vi "ep_Flicker Aggregation PLT (1ch).vi"(0 "flicker Pst":dbl, 1 "restart (F)":bool, 5 "Pst flicker time":timestamp) -> (4 "flicker Plt":dbl, 6 "Plt flicker time":timestamp, 15 "data valid?":bool)   [LabVIEW 2011, in "NI_EP_Power Quality.lvlib"]
uses:
  <vilib>/addons/Electrical Power/PQ/NI_EP_Power Quality.lvlib
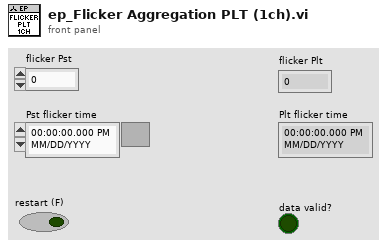
[diagram p1: front panel]
types:
  T1 = typedef "LVDateTimeRec.ctl" = cluster{"fractional second":dbl, "second":i32, "minute":i32, "hour":i32, "day of month":i32, "month":i32, "year":i32, "day of week":i32, "day of year":i32, "DST":i32}
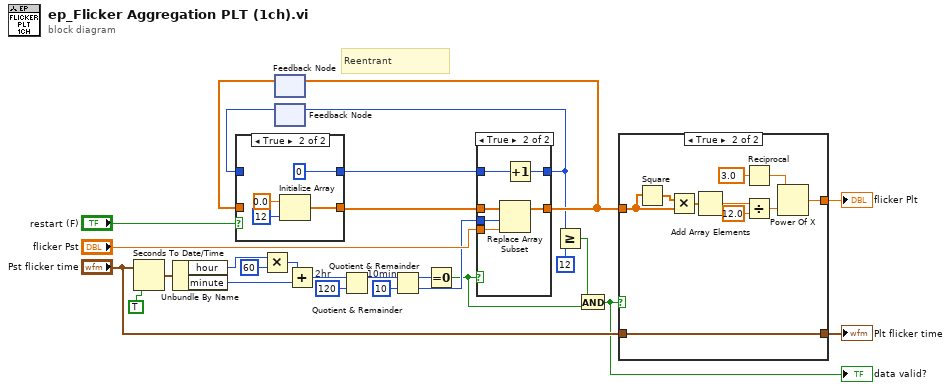
[diagram p0: block diagram]
diagram:
  w15 = 10  # 10min
  w17 = 120  # 2hr
  # "Reentrant"
  n1 = Seconds To Date/Time(time stamp (now)="Pst flicker time", to UTC (F)=TRUE) -> (date time rec=w23:T1)
  n2 = Unbundle By Name(w23) -> ("hour"=w22:i32, "minute"=w19:i32)
  n3 = Multiply(x=w22, y=60) -> (x*y=w20:i32)
  n4 = feedback #1() -> (w26:dbl[])  [unwired: 1 in]
  n5 = feedback #2() -> (w25:i32)  [unwired: 1 in]
  n6 = case shown="True" "restart (F)" {
    tunnel: [w29 w31] -> w12
    tunnel: w26 -> [w29 _]
    tunnel: [w28 0] -> w11
    tunnel: w25 -> [w28 _]
    frame False {
    }
    frame True {
      n7 = Initialize Array(0.0 ("element"), 12 ("dimension size")) -> (w31:dbl[])
    }
  }
  n8 = Add(x=w20, y=w19) -> (x+y=w18:i32)
  n9 = Quotient & Remainder(x=w18, y=w17) -> (x-y*floor(x/y)=w16:i32)  [unwired: 1 out]
  n10 = Quotient & Remainder(x=w16, y=w15) -> (x-y*floor(x/y)=w10:i32, floor(x/y)=w13:i32)
  n11 = Equal To 0?(x=w10) -> (x = 0?=w5:bool)
  n12 = case shown="True" w5 {
    tunnel: "flicker Pst" -> [_ w41]
    tunnel: w13 -> [_ w40]
    tunnel: [w34 w39] -> w9
    tunnel: w12 -> [w34 w38]
    tunnel: [w35 w37] -> w7
    tunnel: w11 -> [w35 w36]
    frame False {
    }
    frame True {
      n13 = Replace Array Subset(array=w38, new element=w41, index=w40) -> (w39:dbl[])
      n14 = Increment(x=w36) -> (x+1=w37:i32)
    }
  }
  n15 = feedback-in #1(w9) -> ()
  n16 = feedback-in #2(w7) -> ()
  n17 = Greater Or Equal?(x=w7, y=12) -> (x >= y?=w4:bool)
  n18 = And(x=w4, y=w5) -> (x .and. y?=w1:bool)
  "data valid?" <- w1
  n19 = case shown="True" w1 {
    tunnel: w9 -> [_ w45]
    tunnel: [_ w43] -> w8
    tunnel: [_ w42] -> w3
    tunnel: "Pst flicker time" -> [_ w42]
    frame False {
    }
    frame True {
      n20 = Square(x=w45) -> (x^2=w48:dbl[])
      n21 = Multiply(x=w48, y=w45) -> (x*y=w47:dbl[])
      n22 = Add Array Elements(numeric array=w47) -> (sum=w51:dbl)
      n23 = Reciprocal(x=3.0) -> (1/x=w44:dbl)
      n24 = Divide(x=w51, y=12.0) -> (x/y=w49:dbl)
      n25 = Power Of X(1:w49, 2:w44) -> (0:w43:dbl)
    }
  }
  "Plt flicker time" <- w3
  "flicker Plt" <- w8
